vi "Loop Status.vi"(8 "error in":errorcluster, 10 "total count":dbl format="%#_6f", 11 "current count":dbl) -> (0 "error out":errorcluster, 1 "Percent Done":dbl(slide) scale=0.0..100.0, 2 "total count":dbl format="%#_6f", 3 "current count":dbl)   [LabVIEW 2017]
panel:
  out "Percent Done":dbl
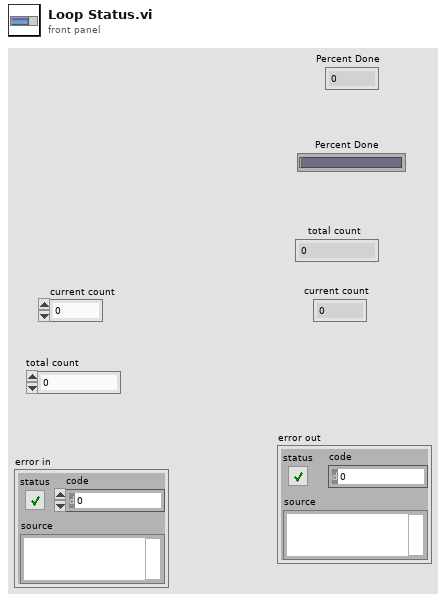
[diagram p1: front panel]
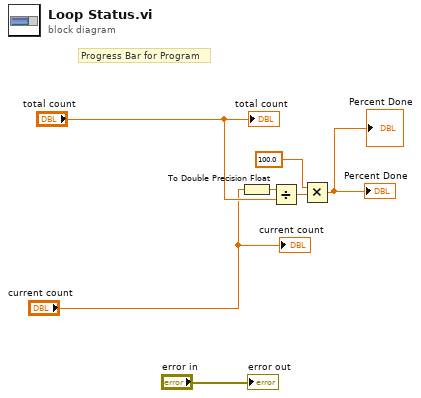
[diagram p0: block diagram]
diagram:
  # "Progress Bar for Program"
  n1 = To Double Precision Float(number="current count") -> (double precision float=w7:dbl)
  n2 = Divide(x=w7, y="total count") -> (x/y=w6:dbl)
  n3 = Multiply(x=100.0, y=w6) -> (x*y=→"Percent Done" →"Percent Done":dbl)
  "total count" <- "total count"
  "current count" <- "current count"
  "error out" <- "error in"
